vi "TrapsMachMitteln-01-17.vi"(0 "FPGA VI Reference In":refnum<k20>, 1 "Traps/MachKoeff2":dbl[](array[numeric]), 2 "Traps/MachKoeff1":dbl[](array[numeric]), 3 "Traps/MachKoeff0":dbl[](array[numeric]), 4 "error in":errorcluster) -> (5 "error out":errorcluster)   [LabVIEW 2010]
uses:
  <vilib>/rvi/interface/nirviReadWriteControl/nirviReadWriteControl.xnode
  C:/Users/HAGAR-IV/Desktop/Zeugs/markus/version feb 2012/FPGA Bitfiles/pertrasgcfpga2_FPGATarget_FPGA-Programm-01_A75D3647.lvbitx
  C:/Users/HAGAR-IV/Desktop/Zeugs/Johnny/pertrasgc fpga/FPGA-Programm-01-17.vi
  <vilib>/rvi/interface/common/niFpgaNodeNameForErrorReporting.ctl
  <vilib>/rvi/errors/niLvFpgaWhatHappensToTopLevelVI.ctl
  GVTrapsMachs.vi
  <vilib>/Utility/error.llb/Error Cluster From Error Code.vi
  <vilib>/rvi/errors/niLvFpgaAdjustHostInterfaceError.vi
  NiFpgaLv.dll
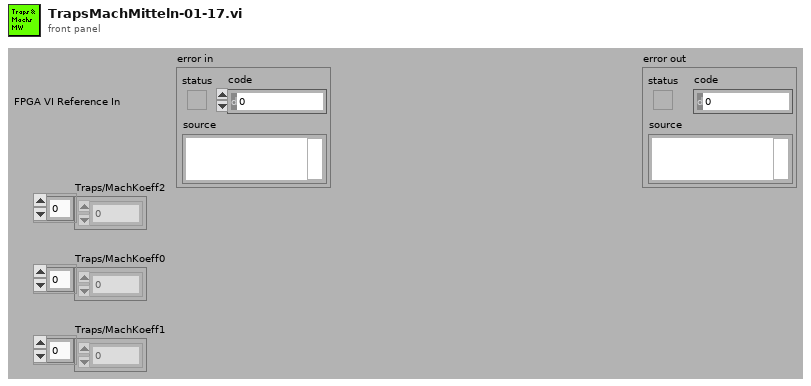
[diagram p1: front panel]
types:
  T1 = typedef "niFpgaNodeNameForErrorReporting.ctl" = enum16{"Open FPGA VI Reference", "Read/Write Control", "Invoke Method: Abort", "Invoke Method: Acknowledge IRQ", "Invoke Method: Download", "Invoke Method: FIFO.Configure", "Invoke Method: FIFO.Read", "Invoke Method: FIFO.Start", "Invoke Method: FIFO.Stop", "Invoke Method: FIFO.Write", "Invoke Method: Reset", "Invoke Method: Run", "Invoke Method: Wait on IRQ", "Close FPGA VI Reference"}
  T2 = typedef "niLvFpgaWhatHappensToTopLevelVI.ctl" = enum16{"top level VI scripted behind XNode", "top level VI inlined behind XNode"}
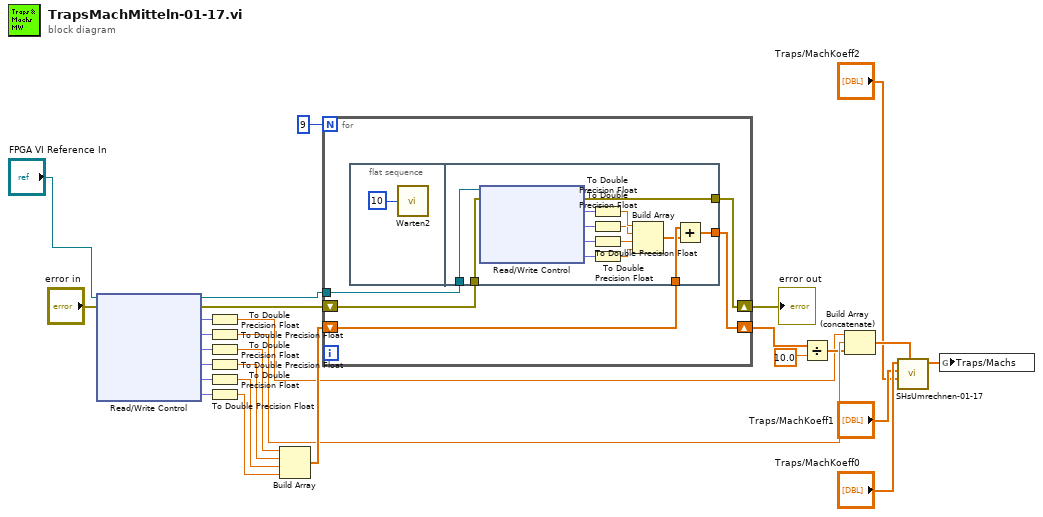
[diagram p0: block diagram]
diagram:
  n1 = xnode "Read/Write Control"("FPGA VI Reference In"="FPGA VI Reference In", "error in"="error in") -> ("FPGA VI Reference Out"=w27:refnum<k20>, "error out"=w3:errorcluster, "MesswertTrap1"=w23:fxp<+/-,27,6>, "PTTrap1"=w22:fxp<+/-,28,7>, "U[V]PreMach1"=w21:fxp<+/-,16,4>, "U[V]PreMach2"=w20:fxp<+/-,16,4>, "U[V]MainMach1"=w19:fxp<+/-,16,4>, "U[V]MainMach2"=w18:fxp<+/-,16,4>)
  n2 = To Double Precision Float(number=w23) -> (double precision float=w10:dbl)
  n3 = To Double Precision Float(number=w22) -> (double precision float=w12:dbl)
  n4 = To Double Precision Float(number=w21) -> (double precision float=w17:dbl)
  n5 = To Double Precision Float(number=w20) -> (double precision float=w16:dbl)
  n6 = To Double Precision Float(number=w19) -> (double precision float=w15:dbl)
  n7 = To Double Precision Float(number=w18) -> (double precision float=w14:dbl)
  n8 = Build Array(w17, w16, w15, w14) -> (w13:dbl[])
  n9 = for {
    N: 9 -> [_]
    tunnel: w27 -> [w32]
    shift-right: [w30] -> w25
    shift-left: w13 -> [w31]
    shift-right: [w28] -> w2
    shift-left: w3 -> [w29]
    n10 = flat-sequence {
      tunnel: w32 -> [w45]
      tunnel: w31 -> [w47]
      tunnel: [w46] -> w30
      tunnel: w29 -> [w35]
      tunnel: [w34] -> w28
      frame #0 {
        n11 = call "Warten2"("Count(mSec)"=u32 10) -> ()  [unwired: 1 out]
      }
      frame #1 {
        n12 = xnode "Read/Write Control"("FPGA VI Reference In"=w45, "error in"=w35) -> ("error out"=w34:errorcluster, "U[V]PreMach1"=w44:fxp<+/-,16,4>, "U[V]PreMach2"=w43:fxp<+/-,16,4>, "U[V]MainMach1"=w42:fxp<+/-,16,4>, "U[V]MainMach2"=w41:fxp<+/-,16,4>)  [unwired: 1 out]
        n13 = To Double Precision Float(number=w44) -> (double precision float=w40:dbl)
        n14 = To Double Precision Float(number=w43) -> (double precision float=w39:dbl)
        n15 = To Double Precision Float(number=w42) -> (double precision float=w38:dbl)
        n16 = To Double Precision Float(number=w41) -> (double precision float=w37:dbl)
        n17 = Build Array(w40, w39, w38, w37) -> (w36:dbl[])
        n18 = Add(x=w47, y=w36) -> (x+y=w46:dbl[])
      }
    }
  }
  "error out" <- w2
  n19 = Divide(x=w25, y=10.0) -> (x/y=w11:dbl[])
  n20 = Build Array (concatenate)(w10, w12, w11) -> (w9:dbl[])
  n21 = call "SHsUmrechnen-01-17.vi"("SpannungenSH[V]"=w9, "Traps/MachKoeff2"="Traps/MachKoeff2", "Traps/MachKoeff1"="Traps/MachKoeff1", "Traps/MachKoeff0"="Traps/MachKoeff0") -> ("TemperaturenSH[°C]"=w5:dbl[])  [unwired: 6 in, 1 out]
  n22 = global write "GVTrapsMachs.vi" "Traps/Machs"(w5) -> ()
